vi "Instrument.Cryostat Class Paths.vi"(7 "instrument":T1) -> (0 "Level Path":path, 1 "Rotator Path":path, 2 "Magnet Path":path, 3 "Temperature Path":path)   [LabVIEW 2016]
uses:
  Typedefs/Instrument--enum.ctl
  AFM Control.lvclass
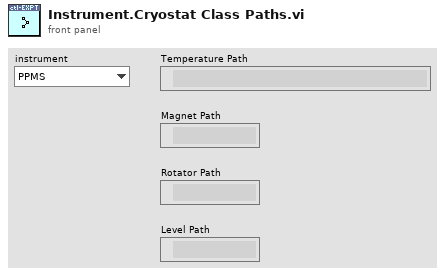
[diagram p1: front panel]
types:
  T1 = typedef "AFM Control.lvclass/Instrument--enum.ctl" = enum16{"PPMS", "PPMS2", "MFP3D", "CYPHER", "THz1", "THz2", "MNK", "CF900", "JEOL", "AGILENT", "EBL"}
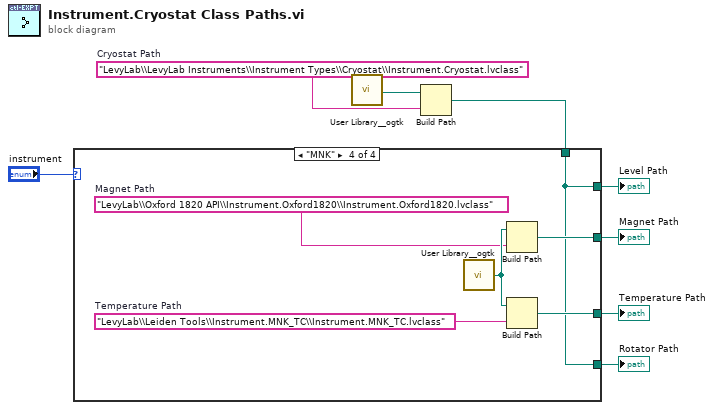
[diagram p0: block diagram]
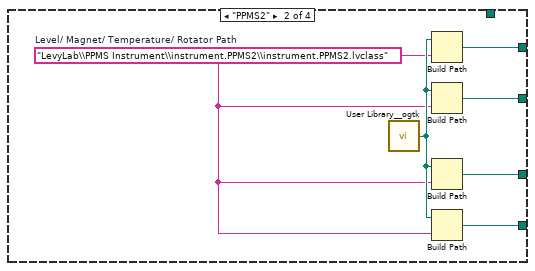
[diagram p3: hidden frame]
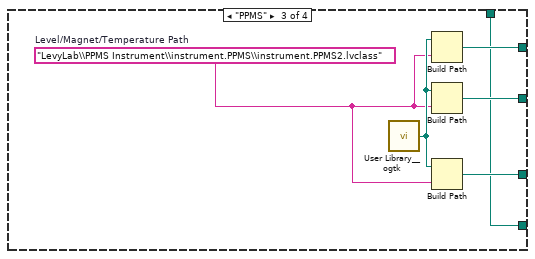
[diagram p4: hidden frame]
diagram:
  w2 = "LevyLab\\LevyLab Instruments\\Instrument Types\\Cryostat\\Instrument.Cryostat.lvclass"  # Cryostat Path
  n1 = call <userlib>:"User Library__ogtk.vi"() -> ("User Library (+ Relative)"=w3:path)  [unwired: 1 in]
  n2 = Build Path(base path=w3, name or relative path=w2) -> (appended path=w1:path)
  n3 = case shown="\"MNK\"" "instrument" {
    tunnel: [w9 w15 w21 w26] -> w5
    tunnel: [w9 w14 w20 w25] -> w4
    tunnel: [w9 w13 w17 w22] -> w7
    tunnel: [w9 w12 w19 w22] -> w6
    tunnel: w1 -> [w9 _ w17 w22]
    frame Default {
    }
    frame "PPMS2" {
      w10 = "LevyLab\\PPMS Instrument\\instrument.PPMS2\\instrument.PPMS2.lvclass"  # Level/ Magnet/ Temperature/ Rotator Path
      n4 = call <userlib>:"User Library__ogtk.vi"() -> ("User Library (+ Relative)"=w11:path)  [unwired: 1 in]
      n5 = Build Path(base path=w11, name or relative path=w10) -> (appended path=w12:path)
      n6 = Build Path(base path=w11, name or relative path=w10) -> (appended path=w14:path)
      n7 = Build Path(base path=w11, name or relative path=w10) -> (appended path=w15:path)
      n8 = Build Path(base path=w11, name or relative path=w10) -> (appended path=w13:path)
    }
    frame "PPMS" {
      w16 = "LevyLab\\PPMS Instrument\\instrument.PPMS\\instrument.PPMS2.lvclass"  # Level/Magnet/Temperature Path
      n9 = call <userlib>:"User Library__ogtk.vi"() -> ("User Library (+ Relative)"=w18:path)  [unwired: 1 in]
      n10 = Build Path(base path=w18, name or relative path=w16) -> (appended path=w19:path)
      n11 = Build Path(base path=w18, name or relative path=w16) -> (appended path=w20:path)
      n12 = Build Path(base path=w18, name or relative path=w16) -> (appended path=w21:path)
    }
    frame "MNK" {
      w23 = "LevyLab\\Oxford 1820 API\\Instrument.Oxford1820\\Instrument.Oxford1820.lvclass"  # Magnet Path
      w27 = "LevyLab\\Leiden Tools\\Instrument.MNK_TC\\Instrument.MNK_TC.lvclass"  # Temperature Path
      n13 = call <userlib>:"User Library__ogtk.vi"() -> ("User Library (+ Relative)"=w24:path)  [unwired: 1 in]
      n14 = Build Path(base path=w24, name or relative path=w23) -> (appended path=w25:path)
      n15 = Build Path(base path=w24, name or relative path=w27) -> (appended path=w26:path)
    }
  }
  "Magnet Path" <- w4
  "Temperature Path" <- w5
  "Rotator Path" <- w7
  "Level Path" <- w6
